vi "Remove Deadband.vi"(9 "Zero Tolerance":dbl=0.05, 10 "Physical Deadband":dbl=0.1, 11 "Output":dbl) -> (3 "Output without deadband":dbl)   [LabVIEW 2012]
panel:
  # "Designed to operate on an output (range -1 to 1) just before setting a motor.\nAnything in the range (-Zero Tolerance, Zero Tolerance) maps to 0.\nOther values are interpolated linearly from -1 at -1 to -Physical Deadband at -Zero Tolerance\nand 1 at 1 to Physical deadband at Zero Tolerance"
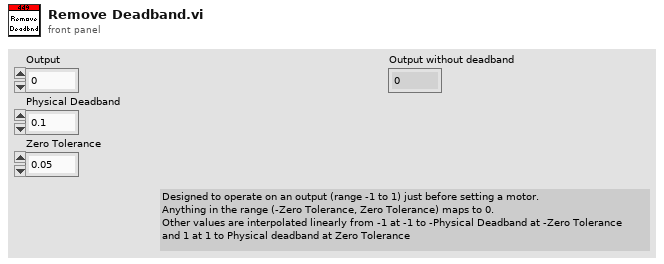
[diagram p1: front panel]
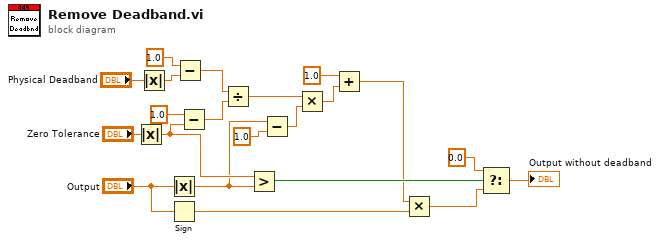
[diagram p0: block diagram]
diagram:
  n1 = Absolute Value(x="Zero Tolerance") -> (abs(x)=w15:dbl)
  n2 = Absolute Value(x="Physical Deadband") -> (abs(x)=w17:dbl)
  n3 = Absolute Value(x="Output") -> (abs(x)=w9:dbl)
  n4 = Sign(1:"Output") -> (0:w3:dbl)
  n5 = Subtract(x=1.0, y=w17) -> (x-y=w12:dbl)
  n6 = Subtract(x=1.0, y=w15) -> (x-y=w13:dbl)
  n7 = Divide(x=w12, y=w13) -> (x/y=w6:dbl)
  n8 = Greater?(x=w15, y=w9) -> (0:w20:bool)
  n9 = Subtract(x=w9, y=1.0) -> (x-y=w7:dbl)
  n10 = Multiply(x=w6, y=w7) -> (x*y=w5:dbl)
  n11 = Add(x=1.0, y=w5) -> (x+y=w4:dbl)
  n12 = Multiply(x=w4, y=w3) -> (x*y=w2:dbl)
  n13 = Select(t=0.0, s=w20, f=w2) -> (s? t:f=→"Output without deadband":dbl)
